vi "getRampTime.vi"(11 "Spinal Column Out":T1={"Red MOT 88 Inputs"={"Active Device"="", "Active Channels"=[], "Waveform Parameters"=[], "Active Phases"=[], "Phase Times"=[], "Trigger Channel"=""}, "6704 Static Voltage Settings"={"Device Name"="", "Values"=[], "Nickname"=[], "Conversion"=[]}, "Instructions"=[], "Red MOT 87 Inputs"={"Active Device"="", "Active Channels"=[], "Waveform Parameters"=[], "Active Phases"=[], "Phase Times"=[], "Trigger Channel"=""}, "ODT Params"={"Waveform Parameters"=[], "Active Phases"=[], "Active Channels"=[], "Phase Times (s)"=[], "Active Device"="", "Trigger Channel"="", "Evaporation Phase"=0.0, "Evaporation Channel"=0.0}, "SR400 Settings"={"Channel A"={"Input"=0, "A Discriminator Level (V)"=0.0, "A Discriminator Slope"=enum."Rising", "A Gate Mode"=enum."CW", "A Gate Delay (s)"=0.0, "A Gate Width (s)"=0.0, "Scan Increment (s)"=0.0}, "Channel B"={"Input"=0, "B Discriminator Level (V)"=0.0, "B Discriminator Slope"=enum."Rising", "B Gate Mode"=enum."CW", "B Gate Delay (s)"=0.0, "B Gate Width (s)"=0.0, "Scan Increment (s)"=0.0}, "Channel T"={"Input"=0, "Trigger Level (V)"=0.0, "Trigger Slope"=enum."Rising", "T Discriminator Slope"=enum."Rising", "T Discriminator Level (V)"=0.0, "Trigger Preset"=0.0}, "N Periods"=0.0, "At N"=enum."Stop", "Counting Mode"=enum."A,B for T Preset", "GPIB Address"="", "Dwell Time (s)"=0.0, "Port 1 Mode"=0, "Port 1 Voltage"=0.0, "Port 1 Scan Increment"=0.0, "Port 2 Voltage"=0.0, "Port 2 Scan Increment"=0.0, "Port 2 Mode"=0, "Counter Toggle"=FALSE, "Pusleblater Settings"={"Loop Start Channel"=0.0, "Loop End Channel"=0.0, "Loop On"=FALSE}}, "Synth Controls"={"Channel Settings"=[], "Active Channels"=[], "COM Port"=""}, "Acquisition Parameters"={"Acquisition Mode"=enum."Reserved (0)", "Trigger Mode"=enum."Internal", "Frame \nTransfer"=FALSE, "Exposure Time (s)"=0.0, "Accumulation Cycle Time (s)"=0.0, "# Accumulations"=0, "# Kinetics"=0, "Kinetic Cycle Time (s)"=0.0, "Horizontal Bin Size"=0, "Vertical Bin Size"=0}, "Scan Parameters"={"Initial Values"=[], "Final Values"=[], "Step Sizes"=[], "Parameters to Change"=[], "Channels to Change"=[], "Number of Parameters to Scan"=0, "Parameter Nickname (no spaces)"=[], "Scan Base Name"="", "Raw_Data Folder"=path "", "ROI Parameters"={"Background Radius"=0.0, "Atom Radius"=0.0, "X Center"=0.0, "Y Center"=0.0}, "Drop Time (ms)"=0.0, "ODT VCA 1 Channel"=0.0, "ODT VCA 2 Channel"=0.0, "Phases To Change"=[], "Scan Pulseblaster Channel With Parameter"={"Change PB Time Toggle"=FALSE, "PB Channel"=0.0, "Parameter Number"=0.0}, "Preserve Waveform\nContinuity"=FALSE, "Generated Array Type"=enum."Custom Array From File", "Principle Quantum #"=0, "Angular Momentum"=enum."s", "Ramp Delay Channel"=0, "ODT Hold Channel"=0, "MCS ROI Min"=0, "MCS ROI Max"=0, "Master Batch Fourth Column"=0.0}, "MCS Parameters"={"Scan Length (Bins)"=0.0, "Dwell Time (s)"=0.0, "Gate Channel Settings"={"Threshold (V)"=0.0, "Edge"=enum."Falling", "Input Impedence"=enum."1k Ohm"}, "Trig Channel Settings"={"Threshold (V)"=0.0, "Edge"=enum."Falling", "Input Impedence"=enum."1k Ohm"}, "Input 1 Settings"={"Threshold (V)"=0.0, "Edge"=enum."Falling", "Input Impedence"=enum."1k Ohm"}, "Input 2 Settings"={"Threshold (V)"=0.0, "Edge"=enum."Falling", "Input Impedence"=enum."1k Ohm"}, "Number of Sweeps"=0, "Number of Sequential Cycles"=0.0, "Number of Sequences"=0.0, "Sweep Preset"=FALSE, "Sequential Mode"=FALSE, "DAC 1 Ramp Settings"={"Ramp Mode"=enum."Fixed", "Ramp Start Value (V)"=0.0, "Ramp Length (Steps)"=0, "Step Width (bins)"=0, "Step Size (V)"=0.0}, "DAC 2 Output (V)"=0.0, "SYNC Output"=enum."40 MHz Clock", "ROI Min"=0, "ROI Max"=0, "Dual MCS Mode"=FALSE, "DAC 2 Toggle"=FALSE, "MCS on/off"=FALSE, "ROI Max 2"=1, "ROI Min 2"=0, "Sum ROI Only"=FALSE, "Use ROI For \nEach Loop"=FALSE}, "PicoScope"={"Channel A Settings"={"Enabled"=FALSE, "Coupling"=0, "Range"=0, "Analogue Offset"=0.0}, "Channel B Settings"={"Enabled"=FALSE, "Coupling"=0, "Range"=0, "Analogue Offset"=0.0}, "Trigger Options"={"Trigger Enabled"=FALSE, "Trigger Source"=enum."Channel A", "Trigger Threshold (-5 to 5 V)"=0.0, "Trigger Slope"=0, "Trigger Delay (ms)"=0.0, "Auto Trigger Time (ms)"=0}, "Pico Scope Inititalization Settings"={"USB Power"=FALSE, "Use Serial Number"=FALSE, "Resolution"=0, "Serial Number"="", "Handle"=0}, "Use PicoScope?"=FALSE, "Acquisition Settings"={"Pre Trigger Time (s)"=0.0, "Post Trigger Time (s)"=0.0, "Resolution (s)"=0.0, "Four Channel Device"=FALSE, "Number of Captures"=0.0}}, "Ramp Delay Settings"={"Subroutine A"=[], "Insert Delays"=FALSE, "Number of loops"=0, "Insert after instruction"=0, "Random"=FALSE, "Initial Delay Time (s)"=0.0, "Final Delay Time (s)"=5e-08, "Delay Step (s)"=5e-08, "Delay Column"=0.0, "Loop Hold Column"=0.0, "Field Ramp Column"=0.0, "Excitation Column"=0.0, "Hold + Delay + Excitation Time"=0.0, "Ascending/Descending"=FALSE}} {"Red MOT 88 Inputs"."Phase Times" format="%.0p"; "Red MOT 87 Inputs"."Phase Times" format="%.0p"; "ODT Params"."Evaporation Channel" min=0.0 max=1.0 step=1.0; "ODT Params"."Evaporation Phase" min=0.0 max=4.0 step=1.0; "ODT Params"."Phase Times (s)" format="%#_6p"; "SR400 Settings"."Port 2 Mode" items=["Scan"=1, "Fixed"=0]; "SR400 Settings"."Port 2 Scan Increment" min=-0.5 max=0.5; "SR400 Settings"."Port 2 Voltage" min=-10.0 max=10.0; "SR400 Settings"."Port 1 Scan Increment" min=-0.5 max=-0.5; "SR400 Settings"."Port 1 Voltage" min=-10.0 max=10.0; "SR400 Settings"."Port 1 Mode" items=["Scan"=1, "Fixed"=0]; "SR400 Settings"."Dwell Time (s)" min=0.002 max=60.0 format="%#_6p"; "SR400 Settings"."N Periods" min=1.0 max=2000.0 step=1.0; "SR400 Settings"."Channel T"."Trigger Preset" min=1.0 max=900000000000.0 format="%#_1e"; "SR400 Settings"."Channel T"."T Discriminator Level (V)" min=-0.3 max=0.3 format="%#_6p"; "SR400 Settings"."Channel T"."Trigger Level (V)" min=-2.0 max=2.0 format="%#_6p"; "SR400 Settings"."Channel T"."Input" items=["10 MHz", "Input 2", "Trig"]; "SR400 Settings"."Channel B"."Scan Increment (s)" min=0.0 max=0.09992 format="%#_6p"; "SR400 Settings"."Channel B"."B Gate Width (s)" min=5e-09 max=0.9992 format="%#_6p"; "SR400 Settings"."Channel B"."B Gate Delay (s)" min=0.0 max=0.9992 format="%#_6p"; "SR400 Settings"."Channel B"."B Discriminator Level (V)" min=-0.3 max=0.3 format="%#_6p"; "SR400 Settings"."Channel B"."Input" items=["Input 2"=2, "Input 1"=1]; "SR400 Settings"."Channel A"."Scan Increment (s)" min=0.0 max=0.09992 format="%#_6p"; "SR400 Settings"."Channel A"."A Gate Width (s)" min=5e-09 max=0.9992 format="%#_6p"; "SR400 Settings"."Channel A"."A Gate Delay (s)" min=0.0 max=0.9992 format="%#_6p"; "SR400 Settings"."Channel A"."A Discriminator Level (V)" min=-0.3 max=0.3 format="%#_6p"; "SR400 Settings"."Channel A"."Input" items=["Input 1", "10 MHz"]; "Acquisition Parameters"."Vertical Bin Size" items=["6"=6, "3"=3, "2"=2, "1"=1]; "Acquisition Parameters"."Horizontal Bin Size" items=["4"=4, "2"=2, "1"=1]; "Acquisition Parameters"."Kinetic Cycle Time (s)" format="%.2f"; "Acquisition Parameters"."# Kinetics" min=1; "Acquisition Parameters"."# Accumulations" min=1; "Acquisition Parameters"."Accumulation Cycle Time (s)" format="%.2f"; "Acquisition Parameters"."Exposure Time (s)" format="%.2f"; "Scan Parameters"."Drop Time (ms)" min=1.0; "Scan Parameters"."Number of Parameters to Scan" min=1; "MCS Parameters"."ROI Max 2" min=1; "MCS Parameters"."ROI Min 2" min=0; "MCS Parameters"."ROI Max" min=1; "MCS Parameters"."ROI Min" min=0; "MCS Parameters"."DAC 2 Output (V)" min=-10.0 max=10.0 step=0.00488; "MCS Parameters"."DAC 1 Ramp Settings"."Step Size (V)" min=0.0 max=10.0 step=0.00244 format="%#_4g"; "MCS Parameters"."DAC 1 Ramp Settings"."Step Width (bins)" min=1; "MCS Parameters"."DAC 1 Ramp Settings"."Ramp Length (Steps)" min=1; "MCS Parameters"."DAC 1 Ramp Settings"."Ramp Start Value (V)" min=0.0 max=10.0 step=0.00244; "MCS Parameters"."Number of Sweeps" min=0 format="%.0p"; "MCS Parameters"."Input 2 Settings"."Threshold (V)" min=-2.5 max=2.5 step=0.001; "MCS Parameters"."Input 1 Settings"."Threshold (V)" min=-2.5 max=2.5 step=0.001; "MCS Parameters"."Trig Channel Settings"."Threshold (V)" min=-2.5 max=2.5 step=0.001; "MCS Parameters"."Gate Channel Settings"."Threshold (V)" min=-2.5 max=2.5 step=0.001; "MCS Parameters"."Dwell Time (s)" min=1e-07 step=2.5e-08 format="%#_6p"; "MCS Parameters"."Scan Length (Bins)" min=64.0 max=524288.0 format="%#_7f"; "PicoScope"."Acquisition Settings"."Resolution (s)" min=8e-09 max=34.36 step=8e-09 format="%#_6p"; "PicoScope"."Acquisition Settings"."Post Trigger Time (s)" min=0.0 format="%#_6p"; "PicoScope"."Acquisition Settings"."Pre Trigger Time (s)" min=0.0 format="%#_6p"; "PicoScope"."Pico Scope Inititalization Settings"."Resolution" items=["8-bit", "12-bit", "14-bit", "15-bit (max. 2 ch.)", "16-bit (max. 1 ch.)"]; "PicoScope"."Trigger Options"."Trigger Slope" items=["Rising"=2, "Falling"=3]; "PicoScope"."Channel B Settings"."Range" items=["10 mV", "20 mV", "50 mV", "100 mV", "200 mV", "500 mV", "1 V", "2 V", "5 V", "10 V", "20 V", "50 V ", "100 V"]; "PicoScope"."Channel B Settings"."Coupling" items=["AC", "DC"]; "PicoScope"."Channel A Settings"."Range" items=["10 mV", "20 mV", "50 mV", "100 mV", "200 mV", "500 mV", "1 V", "2 V", "5 V", "10 V", "20 V", "50 V ", "100 V"]; "PicoScope"."Channel A Settings"."Coupling" items=["AC", "DC"]; "Ramp Delay Settings"."Insert after instruction" min=0; "Ramp Delay Settings"."Delay Step (s)" min=5e-08 format="%#_6p"; "Ramp Delay Settings"."Final Delay Time (s)" min=5e-08 format="%#_6p"; "Ramp Delay Settings"."Initial Delay Time (s)" min=5e-08 format="%#_6p"; "Ramp Delay Settings"."Subroutine A"."Time (s)" min=5e-08 format="%.3p"; "Ramp Delay Settings"."Subroutine A"."Op Code" items=["Continue", "Stop", "Loop", "End Loop", "JSR", "RTS", "Branch", "Long Delay", "Wait"]; "Ramp Delay Settings"."Subroutine A"."Instruct Data" format="%.0p"}) -> (3 "Ramp Time":dbl)   [LabVIEW 2013]
uses:
  2015.06.22_Rydberg_ExpControl/Controls/Spinal Column/spinal_column.ctl
  6733_Red_MOT/6733_control_panel.ctl
  6733_Red_MOT/6733_waveform_parameter_array.ctl
  6733_Red_MOT/6733_waveform_item.ctl
  6733_Red_MOT/6733_voltage_conversions.ctl
  Controls/6704/6704_static_voltages_control.ctl
  Controls/6704/static_voltage_conversions.ctl
  testing ground/6221 arb waveforms/6221_panel.ctl
  testing ground/6221 arb waveforms/6221_waveform_param.ctl
  Controls/SR400/SR400.ctl
  Controls/SR400/Channel A/channelA.ctl
  Controls/SR400/Channel A/channelA_inputs.ctl
  Controls/SR400/discrim_slope.ctl
  Controls/SR400/gate_mode.ctl
  Controls/SR400/Channel B/channelB.ctl
  Controls/SR400/Channel B/inputsB.ctl
  Controls/SR400/Channel T/channelT.ctl
  Controls/SR400/Channel T/inputsT.ctl
  Controls/Synth_409b/Synth_controls.ctl
  Controls/Synth_409b/synth_channel.ctl
  testing ground/AndorCamera/camera_controls.ctl
  testing ground/CameraTest/System Files/user.lib/atmcd32d.llb/AcquisitionMode_mode typedef.ctl
  testing ground/CameraTest/System Files/user.lib/atmcd32d.llb/TriggerMode_mode typedef.ctl
  Controls/ScanParameters/ScanParametersPanel.ctl
  Controls/ScanParameters/ParameterToChange.ctl
  Controls/ScanParameters/ROI_set.ctl
  Controls/ScanParameters/ScanPBandParam.ctl
  Controls/MCS/mcs_control_panel.ctl
  2015.07.19_Rydberg_ExpControl/Controls/MCS/mcs_channel.ctl
  Controls/MCS/ramp_control.ctl
  Controls/PicoScope/pico_control_panel.ctl
  Controls/PicoScope/pico_channel_settings.ctl
  Controls/PicoScope/pico_trigger.ctl
  Controls/PicoScope/pico_init_settings.ctl
  Controls/PulseBlaster/delay_control_2..ctl
panel:
  # "(0) 689 Center Freq"
  # "(1) 689 Dither Amp"
  # "(2) 689 Power Lock"
  # "(3) Red MOT Field Grad"
  # "(0) 689 Center Freq"
  # "(1) 689 Dither Amp"
  # "(2) 689 Power Lock"
  # "(3) Red MOT Field Grad"
  # "Select a PB Channel to set with a phase time\nfor evaporation or whatever"
  # "1"
  # "2"
  # "3"
  # "4"
  # "5"
  # "6"
  # "7"
  # "8"
  # "9"
  # "10"
  # "11"
  # "12"
  # "13"
  # "14"
  # "15"
  # "16"
  # "17"
  # "18"
  # "19"
  # "20"
  # "21"
  # "22"
  # "23"
  # "24"
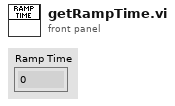
[diagram p1: front panel]
types:
  T1 = typedef "spinal_column.ctl" = cluster{"Red MOT 88 Inputs":T2, "6704 Static Voltage Settings":T6, "Instructions":cluster{"Instruct Data":i32, "Op Code":i32, "Flags":bool[], "Comments":string, "Time (s)":dbl}[], "Red MOT 87 Inputs":T2, "ODT Params":T8, "SR400 Settings":T10, "Synth Controls":T19, "Acquisition Parameters":T21, "Scan Parameters":T24, "MCS Parameters":T28, "PicoScope":T31, "Ramp Delay Settings":T35}
  T2 = typedef "6733_control_panel.ctl" = cluster{"Active Device":string, "Active Channels":bool[], "Waveform Parameters":T3, "Active Phases":bool[], "Phase Times":dbl[], "Trigger Channel":tag}
  T3 = typedef "6733_waveform_parameter_array.ctl" = T4[][]
  T4 = typedef "6733_waveform_item.ctl" = cluster{"Functional Form":enum16{"Polynomial", "Exponential"}, "Start Voltage":dbl, "End Voltage":dbl, "Degree":i8, "Nickname":string, "Conversion":T5}
  T5 = typedef "6733_voltage_conversions.ctl" = enum16{"B Field Grad (G/cm)", "Red AOM Center Freq (MHz)", "Red Dither Pk(kHz)", "Red Power (mW)", "Volts"}
  T6 = typedef "6704_static_voltages_control.ctl" = cluster{"Device Name":string, "Values":dbl[], "Nickname":string[], "Conversion":T7[]}
  T7 = typedef "static_voltage_conversions.ctl" = enum16{"Volts", "ODT Power Lock (W)", "Sat Abs Detuning (MHz)", "Blue Mot Power Lock (mW)"}
  T8 = typedef "6221_panel.ctl" = cluster{"Waveform Parameters":T9[][], "Active Phases":bool[], "Active Channels":bool[], "Phase Times (s)":dbl[], "Active Device":string, "Trigger Channel":tag, "Evaporation Phase":dbl, "Evaporation Channel":dbl}
  T9 = typedef "6221_waveform_param.ctl" = cluster{"Initial Value":dbl, "Final Value":dbl, "Tau":dbl, "Eta":dbl, "Nickname":string, "Enum":enum16{"Volts to Volts", "Power Law", "Evaporation Formula"}}
  T10 = typedef "SR400.ctl" = cluster{"Channel A":T11, "Channel B":T15, "Channel T":T17, "N Periods":dbl, "At N":enum16{"Stop", "Start"}, "Counting Mode":enum16{"A,B for T Preset", "A-B for T Preset", "A+B for T Preset"}, "GPIB Address":string, "Dwell Time (s)":dbl, "Port 1 Mode":i32, "Port 1 Voltage":dbl, "Port 1 Scan Increment":dbl, "Port 2 Voltage":dbl, "Port 2 Scan Increment":dbl, "Port 2 Mode":i32, "Counter Toggle":bool, "Pusleblater Settings":cluster{"Loop Start Channel":dbl, "Loop End Channel":dbl, "Loop On":bool}}
  T11 = typedef "channelA.ctl" = cluster{"Input":T12, "A Discriminator Level (V)":dbl, "A Discriminator Slope":T13, "A Gate Mode":T14, "A Gate Delay (s)":dbl, "A Gate Width (s)":dbl, "Scan Increment (s)":dbl}
  T12 = typedef "channelA_inputs.ctl" = u16
  T13 = typedef "discrim_slope.ctl" = enum16{"Rising", "Falling"}
  T14 = typedef "gate_mode.ctl" = enum16{"CW", "Fixed", "Scan"}
  T15 = typedef "channelB.ctl" = cluster{"Input":T16, "B Discriminator Level (V)":dbl, "B Discriminator Slope":T13, "B Gate Mode":T14, "B Gate Delay (s)":dbl, "B Gate Width (s)":dbl, "Scan Increment (s)":dbl}
  T16 = typedef "inputsB.ctl" = u16
  T17 = typedef "channelT.ctl" = cluster{"Input":T18, "Trigger Level (V)":dbl, "Trigger Slope":T13, "T Discriminator Slope":T13, "T Discriminator Level (V)":dbl, "Trigger Preset":dbl}
  T18 = typedef "inputsT.ctl" = u16
  T19 = typedef "Synth_controls.ctl" = cluster{"Channel Settings":T20[], "Active Channels":bool[], "COM Port":refnum<visa-resource-name>}
  T20 = typedef "synth_channel.ctl" = cluster{"Voltage (Pk-Pk) ":dbl, "Frequency (MHz)":dbl, "Phase (deg)":dbl, "Nickname":string}
  T21 = typedef "camera_controls.ctl" = cluster{"Acquisition Mode":T22, "Trigger Mode":T23, "Frame \nTransfer":bool, "Exposure Time (s)":sgl, "Accumulation Cycle Time (s)":sgl, "# Accumulations":i32, "# Kinetics":i32, "Kinetic Cycle Time (s)":sgl, "Horizontal Bin Size":i32, "Vertical Bin Size":i32}
  T22 = typedef "AcquisitionMode_mode typedef.ctl" = enum16{"Reserved (0)", "Single Scan", "Accumulate", "Kinetics", "Fast Kinetics", "Run Till Abort", "Reserved (6)", "Reserved (7)", "Reserved (8)", "Time Delayed Integration"}
  T23 = typedef "TriggerMode_mode typedef.ctl" = enum16{"Internal", "External", "N/A (2)", "N/A (3)", "N/A (4)", "N/A (5)", "External Start", "External Exposure (Bulb)", "N/A (8)", "External FVB EM", "Software", "N/A (11)", "External Charge Shifting"}
  T24 = typedef "ScanParametersPanel.ctl" = cluster{"Initial Values":dbl[], "Final Values":dbl[], "Step Sizes":dbl[], "Parameters to Change":T25[], "Channels to Change":dbl[], "Number of Parameters to Scan":i32, "Parameter Nickname (no spaces)":string[], "Scan Base Name":string, "Raw_Data Folder":path, "ROI Parameters":T26, "Drop Time (ms)":dbl, "ODT VCA 1 Channel":dbl, "ODT VCA 2 Channel":dbl, "Phases To Change":dbl[], "Scan Pulseblaster Channel With Parameter":T27, "Preserve Waveform\nContinuity":bool, "Generated Array Type":enum16{"Custom Array From File", "Default (old way)"}, "Principle Quantum #":i32, "Angular Momentum":enum16{"s", "p", "d", "f", "g", "h"}, "Ramp Delay Channel":i32, "ODT Hold Channel":i32, "MCS ROI Min":i32, "MCS ROI Max":i32, "Master Batch Fourth Column":dbl}
  T25 = typedef "ParameterToChange.ctl" = enum16{"Delay single delay time", "Dummy Variable", "Delay Exposure", "PB Loops", "Number of Delay Loops", "Subroutine A Time", "Subroutine B Time", "Synth Amplitude", "Synth Frequency", "Synth Phase", "ODT Params Phase Time", "ODT Params Tau", "ODT Params Final Voltage", "ODT Params Initial Voltage", "ODT Params Eta", "Red Mot 88 Phase Time", "Red Mot 87 Phase Time", "Red Mot 88 Final Voltage", "Red Mot 88 Initial Voltage", "Red Mot 87 Final Voltage", "Red Mot 87 Initial Voltage", "PulseBlaster", "Static Voltage"}
  T26 = typedef "ROI_set.ctl" = cluster{"Background Radius":dbl, "Atom Radius":dbl, "X Center":dbl, "Y Center":dbl}
  T27 = typedef "ScanPBandParam.ctl" = cluster{"Change PB Time Toggle":bool, "PB Channel":dbl, "Parameter Number":dbl}
  T28 = typedef "mcs_control_panel.ctl" = cluster{"Scan Length (Bins)":dbl, "Dwell Time (s)":dbl, "Gate Channel Settings":T29, "Trig Channel Settings":T29, "Input 1 Settings":T29, "Input 2 Settings":T29, "Number of Sweeps":i32, "Number of Sequential Cycles":dbl, "Number of Sequences":dbl, "Sweep Preset":bool, "Sequential Mode":bool, "DAC 1 Ramp Settings":T30, "DAC 2 Output (V)":dbl, "SYNC Output":enum16{"40 MHz Clock", "Gate Disc Signal", "Trigger Disc Signal", "Counter 1 Disc Signal", "Counter 2 Disc Signal", "Definitely Not Used", "Not Used", "1 kHz Signal", "Also Not Used", "MCS On/Off", "End of Time Bin", "Ramp Increment Trig", "Step Count Trigger", "'GO'-Line", "Ramp Down Trigger", "Logic 1"}, "ROI Min":i32, "ROI Max":i32, "Dual MCS Mode":bool, "DAC 2 Toggle":bool, "MCS on/off":bool, "ROI Max 2":i32, "ROI Min 2":i32, "Sum ROI Only":bool, "Use ROI For \nEach Loop":bool}
  T29 = typedef "mcs_channel.ctl" = cluster{"Threshold (V)":dbl, "Edge":enum16{"Falling", "Rising"}, "Input Impedence":enum16{"1k Ohm", "50 Ohm"}}
  T30 = typedef "ramp_control.ctl" = cluster{"Ramp Mode":enum16{"Fixed", "Triangle", "Sawtooth"}, "Ramp Start Value (V)":dbl, "Ramp Length (Steps)":i32, "Step Width (bins)":i32, "Step Size (V)":dbl}
  T31 = typedef "pico_control_panel.ctl" = cluster{"Channel A Settings":T32, "Channel B Settings":T32, "Trigger Options":T33, "Pico Scope Inititalization Settings":T34, "Use PicoScope?":bool, "Acquisition Settings":cluster{"Pre Trigger Time (s)":dbl, "Post Trigger Time (s)":dbl, "Resolution (s)":dbl, "Four Channel Device":bool, "Number of Captures":dbl}}
  T32 = typedef "pico_channel_settings.ctl" = cluster{"Enabled":bool, "Coupling":i16, "Range":u16, "Analogue Offset":sgl}
  T33 = typedef "pico_trigger.ctl" = cluster{"Trigger Enabled":bool, "Trigger Source":enum16{"Channel A", "Channel B", "Channel C", "Channel D", "Ext."}, "Trigger Threshold (-5 to 5 V)":dbl, "Trigger Slope":u16, "Trigger Delay (ms)":dbl, "Auto Trigger Time (ms)":i16}
  T34 = typedef "pico_init_settings.ctl" = cluster{"USB Power":bool, "Use Serial Number":bool, "Resolution":i32, "Serial Number":string, "Handle":i16}
  T35 = typedef "delay_control_2..ctl" = cluster{"Subroutine A":cluster{"Instruct Data":i32, "Op Code":i32, "Flags":bool[], "Comments":string, "Time (s)":dbl}[], "Insert Delays":bool, "Number of loops":i32, "Insert after instruction":i32, "Random":bool, "Initial Delay Time (s)":dbl, "Final Delay Time (s)":dbl, "Delay Step (s)":dbl, "Delay Column":dbl, "Loop Hold Column":dbl, "Field Ramp Column":dbl, "Excitation Column":dbl, "Hold + Delay + Excitation Time":dbl, "Ascending/Descending":bool}
  T36 = cluster{"Instruct Data":i32, "Op Code":i32, "Flags":bool[], "Comments":string, "Time (s)":dbl}[]
  T37 = cluster{"Instruct Data":i32, "Op Code":i32, "Flags":bool[], "Comments":string, "Time (s)":dbl}
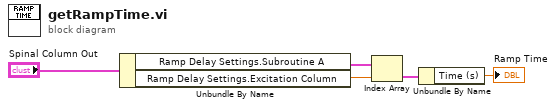
[diagram p0: block diagram]
diagram:
  n1 = Unbundle By Name("Spinal Column Out") -> ("Ramp Delay Settings.Subroutine A"=w4:T36, "Ramp Delay Settings.Excitation Column"=w3:dbl)
  n2 = Index Array(array=w4, index=w3) -> (element=w2:T37)
  n3 = Unbundle By Name(w2) -> ("Time (s)"=→"Ramp Time":dbl)
